vi "Get_New_Image_Coords_after_Scale.vi"(4 "Image Type":T1=4 items=["Grayscale (U8)", "Grayscale (I16)", "Grayscale (SGL)", "Complex (CSG)", "RGB (U32)", "HSL (U32)", "RGB (U64)", "Grayscale (U16)"], 6 "Modified":T2, 7 "Scale":sgl, 8 "Error In":errorcluster, 9 "Shift(W)":sgl, 10 "Shift(H)":sgl, 11 "Image In":T2) -> (0 "Error Out":errorcluster, 2 "New Coords after zoom":sgl[](array[numeric]) format="%.2f", 3 "Image out":T2)   [LabVIEW 2020]
uses:
  <vilib>/vision/Image Controls.llb/IMAQ Image.ctl
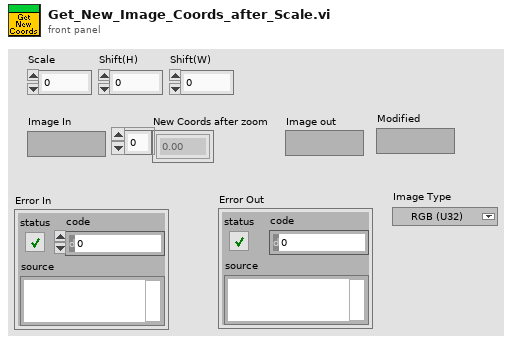
[diagram p1: front panel]
types:
  T1 = typedef "Image Type" = u32
  T2 = typedef "IMAQ Image.ctl" = refnum<image>
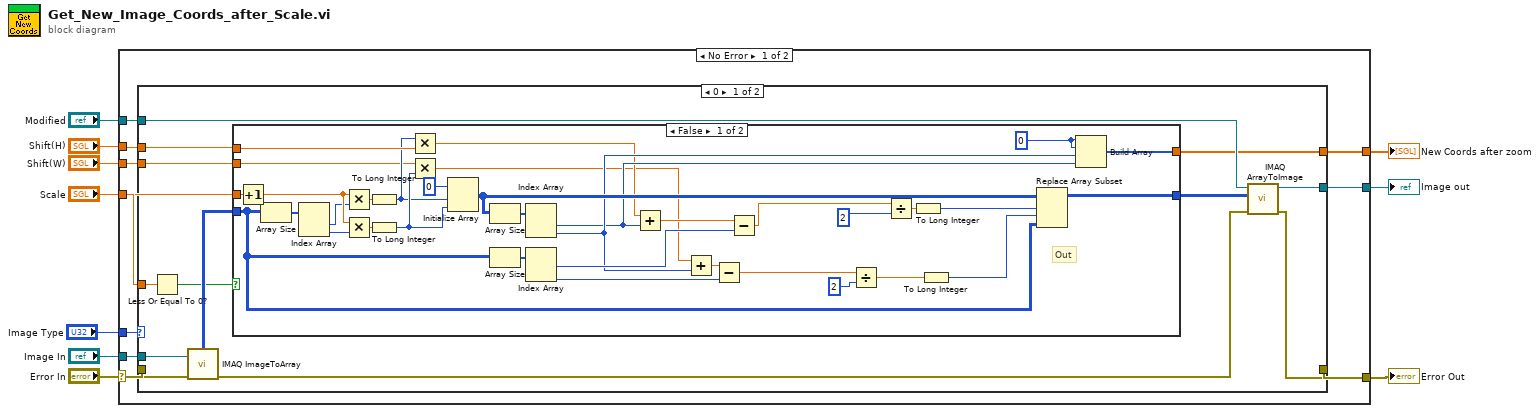
[diagram p0: block diagram]
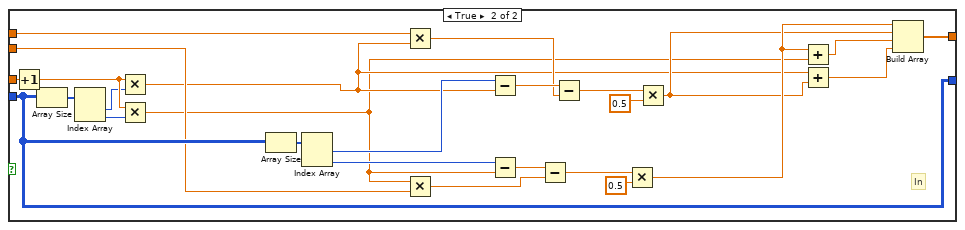
[diagram p2: hidden frame]
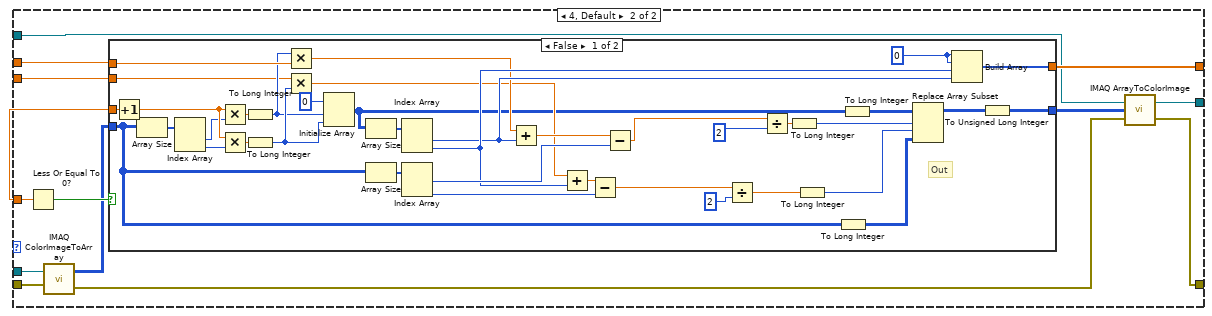
[diagram p3: hidden frame]
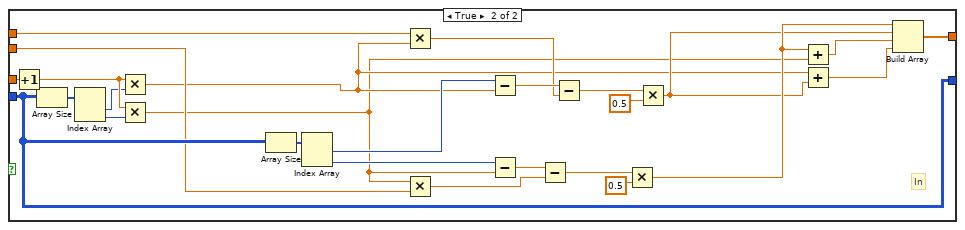
[diagram p4: hidden frame]
diagram:
  n1 = case shown="No Error" "Error In" {
    selector: "Error In" -> [w19 w173]
    tunnel: [w20 w172] -> w5
    tunnel: "Image In" -> [w17 w172]
    tunnel: [w18 w173] -> w8
    tunnel: "Scale" -> [w16 _]
    tunnel: "Shift(H)" -> [w15 _]
    tunnel: [w12 _] -> w4
    tunnel: "Shift(W)" -> [w14 _]
    tunnel: "Modified" -> [w13 _]
    tunnel: "Image Type" -> [w11 _]
    frame No Error {
      n2 = case shown="0" w11 {
        tunnel: [w33 w97] -> w20
        tunnel: w19 -> [w32 w100]
        tunnel: [w30 w95] -> w18
        tunnel: w17 -> [w28 w102]
        tunnel: w16 -> [w27 w107]
        tunnel: w15 -> [w26 w106]
        tunnel: w14 -> [w25 w105]
        tunnel: w13 -> [w24 w98]
        tunnel: [w23 w104] -> w12
        frame 0 {
          n3 = Less Or Equal To 0?(x=w27) -> (x <= 0?=w22:bool)
          n4 = call "IMAQ ImageToArray"("error in (no error)"=w32, "Image"=w28) -> ("error out"=w31:errorcluster, "Image Pixels (U8)"=w29:u8[][])  [unwired: 2 in, 3 out]
          n5 = case shown="False" w22 {
            tunnel: w29 -> [w55 w75]
            tunnel: w27 -> [w53 w87]
            tunnel: w26 -> [w50 w74]
            tunnel: w25 -> [w45 w73]
            tunnel: [w44 w75] -> w21
            tunnel: [w41 w82] -> w23
            frame False {
              w36 = 0 ("element")
              # "Out"
              n6 = Increment(x=w53) -> (x+1=w54:sgl)
              n7 = Array Size(array=w55) -> (size(s)=w67:i32[])
              n8 = Index Array(array=w67) -> (element #1=w52:i32, element #2=w51:i32)  [unwired: 2 in]
              n9 = Multiply(x=w54, y=w52) -> (x*y=w65:sgl)
              n10 = Multiply(x=w54, y=w51) -> (x*y=w66:sgl)
              n11 = To Long Integer(number=w65) -> (32bit integer=w46:i32)
              n12 = To Long Integer(number=w66) -> (32bit integer=w47:i32)
              n13 = Multiply(x=w46, y=w50) -> (x*y=w39:sgl)
              n14 = Multiply(x=w45, y=w47) -> (x*y=w38:sgl)
              n15 = Initialize Array(u8 0 ("dimension size"), w46, w47) -> (w64:u8[][])
              n16 = Array Size(array=w64) -> (size(s)=w63:i32[])
              n17 = Array Size(array=w55) -> (size(s)=w62:i32[])
              n18 = Index Array(array=w63) -> (element #1=w42:i32, element #2=w43:i32)  [unwired: 2 in]
              n19 = Index Array(array=w62) -> (element #1=w61:i32, element #2=w56:i32)  [unwired: 2 in]
              n20 = Add(x=w39, y=w42) -> (x+y=w49:sgl)
              n21 = Add(x=w38, y=w43) -> (x+y=w48:sgl)
              n22 = Subtract(x=w48, y=w56) -> (x-y=w57:sgl)
              n23 = Subtract(x=w49, y=w61) -> (x-y=w60:sgl)
              n24 = Divide(x=w57, y=2 ("x")) -> (x/y=w40:sgl)
              n25 = Divide(x=w60, y=2 ("x")) -> (x/y=w37:sgl)
              n26 = To Long Integer(number=w37) -> (32bit integer=w35:i32)
              n27 = To Long Integer(number=w40) -> (32bit integer=w34:i32)
              n28 = Replace Array Subset(array=w64, new element=w55, index (row)=w35, index (col)=w34) -> (w44:u8[][])
              n29 = Build Array(w36, w36, w43, w42) -> (w41:i32[])
            }
            frame True {
              # "In"
              n30 = Increment(x=w87) -> (x+1=w88:sgl)
              n31 = Array Size(array=w75) -> (size(s)=w94:i32[])
              n32 = Index Array(array=w94) -> (element #1=w86:i32, element #2=w85:i32)  [unwired: 2 in]
              n33 = Multiply(x=w88, y=w86) -> (x*y=w70:sgl)
              n34 = Multiply(x=w88, y=w85) -> (x*y=w69:sgl)
              n35 = Array Size(array=w75) -> (size(s)=w93:i32[])
              n36 = Index Array(array=w93) -> (element #1=w72:i32, element #2=w71:i32)  [unwired: 2 in]
              n37 = Multiply(x=w74, y=w70) -> (x*y=w79:sgl)
              n38 = Multiply(x=w69, y=w73) -> (x*y=w77:sgl)
              n39 = Subtract(x=w72, y=w70) -> (x-y=w92:sgl)
              n40 = Subtract(x=w71, y=w69) -> (x-y=w89:sgl)
              n41 = Subtract(x=w89, y=w77) -> (x-y=w78:sgl)
              n42 = Subtract(x=w92, y=w79) -> (x-y=w80:sgl)
              n43 = Multiply(x=w78, y=sgl 0.5 ("x")) -> (x*y=w81:sgl)
              n44 = Multiply(x=w80, y=sgl 0.5 ("x")) -> (x*y=w76:sgl)
              n45 = Add(x=w81, y=w69) -> (x+y=w84:sgl)
              n46 = Add(x=w70, y=w76) -> (x+y=w83:sgl)
              n47 = Build Array(w81, w76, w84, w83) -> (w82:sgl[])
            }
          }
          n48 = call "IMAQ ArrayToImage"("error in (no error)"=w31, "Image Pixels (U8)"=w21, "Image"=w24) -> ("error out"=w30:errorcluster, "Image Out"=w33:T2)  [unwired: 7 in]
        }
        frame 4, Default {
          n49 = Less Or Equal To 0?(x=w107) -> (x <= 0?=w103:bool)
          n50 = call "IMAQ ColorImageToArray"("Image"=w102, "error in (no error)"=w100) -> ("Image Pixels (U32)"=w101:u32[][], "error out"=w96:errorcluster)  [unwired: 2 in, 1 out]
          n51 = case shown="False" w103 {
            tunnel: w101 -> [w111 w152]
            tunnel: w107 -> [w132 w164]
            tunnel: w106 -> [w129 w151]
            tunnel: w105 -> [w124 w150]
            tunnel: [w108 w152] -> w99
            tunnel: [w121 w159] -> w104
            frame False {
              w116 = 0 ("element")
              # "Out"
              n52 = Increment(x=w132) -> (x+1=w133:sgl)
              n53 = Array Size(array=w111) -> (size(s)=w144:i32[])
              n54 = Index Array(array=w144) -> (element #1=w131:i32, element #2=w130:i32)  [unwired: 2 in]
              n55 = Multiply(x=w133, y=w131) -> (x*y=w142:sgl)
              n56 = Multiply(x=w133, y=w130) -> (x*y=w143:sgl)
              n57 = To Long Integer(number=w142) -> (32bit integer=w125:i32)
              n58 = To Long Integer(number=w143) -> (32bit integer=w126:i32)
              n59 = Multiply(x=w125, y=w129) -> (x*y=w119:sgl)
              n60 = Multiply(x=w124, y=w126) -> (x*y=w118:sgl)
              n61 = Initialize Array(u8 0 ("dimension size"), w125, w126) -> (w113:u8[][])
              n62 = Array Size(array=w113) -> (size(s)=w141:i32[])
              n63 = Array Size(array=w111) -> (size(s)=w140:i32[])
              n64 = Index Array(array=w141) -> (element #1=w122:i32, element #2=w123:i32)  [unwired: 2 in]
              n65 = Index Array(array=w140) -> (element #1=w139:i32, element #2=w134:i32)  [unwired: 2 in]
              n66 = Add(x=w119, y=w122) -> (x+y=w128:sgl)
              n67 = Add(x=w118, y=w123) -> (x+y=w127:sgl)
              n68 = Subtract(x=w127, y=w134) -> (x-y=w135:sgl)
              n69 = Subtract(x=w128, y=w139) -> (x-y=w138:sgl)
              n70 = Divide(x=w135, y=2 ("x")) -> (x/y=w120:sgl)
              n71 = Divide(x=w138, y=2 ("x")) -> (x/y=w117:sgl)
              n72 = To Long Integer(number=w117) -> (32bit integer=w115:i32)
              n73 = To Long Integer(number=w120) -> (32bit integer=w114:i32)
              n74 = To Long Integer(number=w111) -> (32bit integer=w110:i32[][])
              n75 = To Long Integer(number=w113) -> (32bit integer=w112:i32[][])
              n76 = Replace Array Subset(array=w112, new element=w110, index (row)=w115, index (col)=w114) -> (w109:i32[][])
              n77 = Build Array(w116, w116, w123, w122) -> (w121:i32[])
              n78 = To Unsigned Long Integer(number=w109) -> (unsigned 32bit integer=w108:u32[][])
            }
            frame True {
              # "In"
              n79 = Increment(x=w164) -> (x+1=w165:sgl)
              n80 = Array Size(array=w152) -> (size(s)=w171:i32[])
              n81 = Index Array(array=w171) -> (element #1=w163:i32, element #2=w162:i32)  [unwired: 2 in]
              n82 = Multiply(x=w165, y=w163) -> (x*y=w147:sgl)
              n83 = Multiply(x=w165, y=w162) -> (x*y=w146:sgl)
              n84 = Array Size(array=w152) -> (size(s)=w170:i32[])
              n85 = Index Array(array=w170) -> (element #1=w149:i32, element #2=w148:i32)  [unwired: 2 in]
              n86 = Multiply(x=w151, y=w147) -> (x*y=w156:sgl)
              n87 = Multiply(x=w146, y=w150) -> (x*y=w154:sgl)
              n88 = Subtract(x=w149, y=w147) -> (x-y=w169:sgl)
              n89 = Subtract(x=w148, y=w146) -> (x-y=w166:sgl)
              n90 = Subtract(x=w166, y=w154) -> (x-y=w155:sgl)
              n91 = Subtract(x=w169, y=w156) -> (x-y=w157:sgl)
              n92 = Multiply(x=w155, y=sgl 0.5 ("x")) -> (x*y=w158:sgl)
              n93 = Multiply(x=w157, y=sgl 0.5 ("x")) -> (x*y=w153:sgl)
              n94 = Add(x=w158, y=w146) -> (x+y=w161:sgl)
              n95 = Add(x=w147, y=w153) -> (x+y=w160:sgl)
              n96 = Build Array(w158, w153, w161, w160) -> (w159:sgl[])
            }
          }
          n97 = call "IMAQ ArrayToColorImage"("Image Pixels (U32)"=w99, "Image"=w98, "error in (no error)"=w96) -> ("Image Out"=w97:T2, "error out"=w95:errorcluster)  [unwired: 2 in]
        }
      }
    }
    frame Error {
    }
  }
  "Image out" <- w5
  "Error Out" <- w8
  "New Coords after zoom" <- w4
